vi "CheckifINorOUTIrregularForceField.vi"(0 "CenPt":dbl[](array[numeric])) -> (7 "DesiredFM_FF":dbl[](array[numeric]), 8 "Current_point":dbl[](array[numeric]), 10 "in":bool)   [LabVIEW 2017]
uses:
  <vilib>/imath/engines/lvmath2/RunTimeEngine/IndexRead/NIMS V(S).vi
  <instcachedir>/0/NIMS V(S)_0488751826AF41519A22953C041130DC.lvgen/NIMS V(S)_0488751826AF41519A22953C041130DC_000.vi
  <vilib>/imathl/engines/lvmath/Functions/Error Handling/Create Error.vi
  <vilib>/imath/engines/lvmath2/RunTimeEngine/VariableToken/NIMS_VariableToken_CondDefined.vi
  <instcachedir>/0/NIMS_VariableToken_CondDefined_6E7F1EE7F80E48298C84CF05BD736261.lvgen/NIMS_VariableToken_CondDefined_6E7F1EE7F80E48298C84CF05BD736261_004.vi
  <vilib>/imath/engines/lvmath/Functions/Error Handling/MergeErrorsWrapper.vi
  <vilib>/imath/engines/lvmath2/RunTimeEngine/NodeEndStatement/NIMS_NodeEndStatement_Output.vi
  <instcachedir>/0/NIMS_NodeEndStatement_Output_53EC0D466D134D7ABD903AC30B43404B.lvgen/NIMS_NodeEndStatement_Output_53EC0D466D134D7ABD903AC30B43404B_001.vi
  <instcachedir>/0/NIMS_NodeEndStatement_Output_53EC0D466D134D7ABD903AC30B43404B.lvgen/NIMS_NodeEndStatement_Output_53EC0D466D134D7ABD903AC30B43404B_005.vi
  <instcachedir>/0/NIMS_NodeEndStatement_Output_53EC0D466D134D7ABD903AC30B43404B.lvgen/NIMS_NodeEndStatement_Output_53EC0D466D134D7ABD903AC30B43404B_010.vi
  <vilib>/imath/engines/lvmath2/RunTimeEngine/ErrorHandling/NIMS_Finalize Error.vi
panel:
  out "z":dbl
  out "y":dbl
  out "x":dbl
  out "c":dbl
  out "b":dbl
  out "a":dbl
  out "value":dbl
  out "FX FY FZ 0 0 0":dbl[](array[numeric])
  out "Fx, Fy, Fz":dbl[](array[numeric])
  out "subarray 2":dbl[](array[numeric])
  out "Desired FM_FF":dbl[](array[numeric])
  # "Inputs"
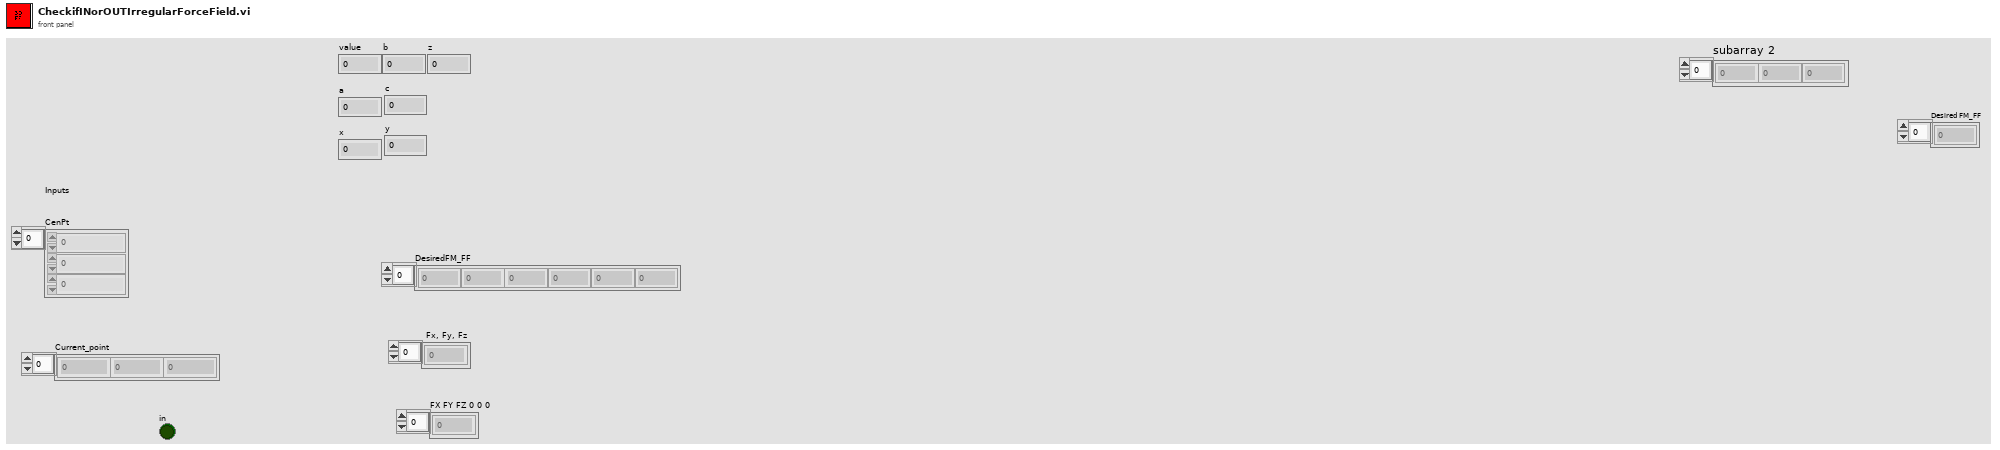
[diagram p1: front panel]
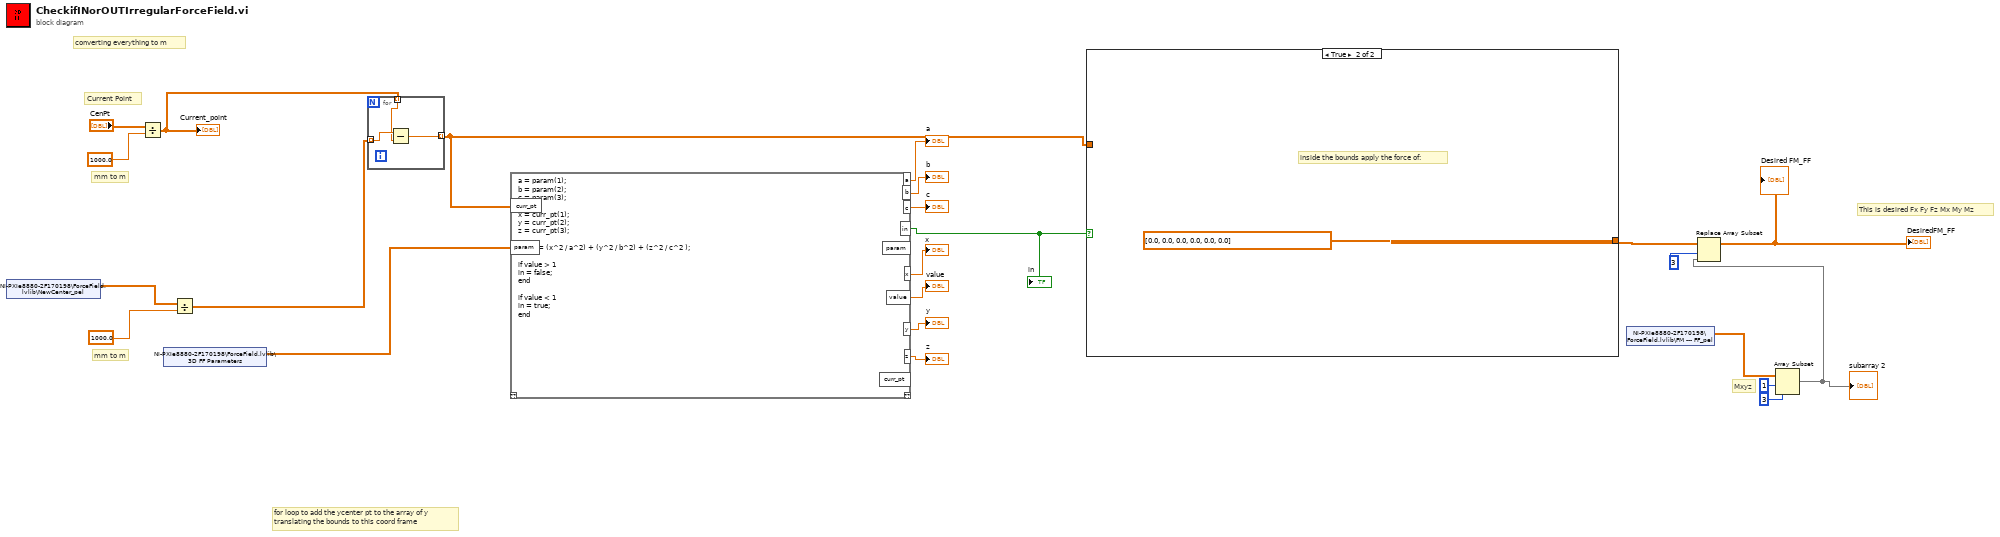
[diagram p0: block diagram]
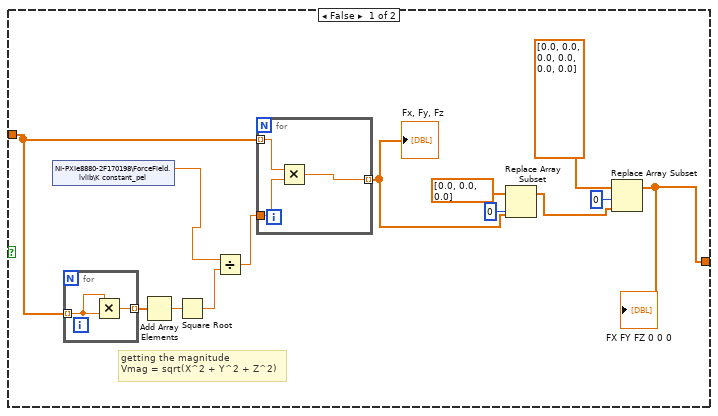
[diagram p2: hidden frame]
diagram:
  # "for loop to add the ycenter pt to the array of y\ntranslating the bounds to this coord frame"
  # "This is desired Fx Fy Fz Mx My Mz"
  # "converting everything to m"
  # "Mxyz"
  # "mm to m"
  # "Current Point"
  # "mm to m"
  n1 = shared-variable "NI-PXIe8880-2F170198\\ForceField.lvlib\\NewCenter_pel"() -> (w9:dbl[])  [unwired: 1 in, 1 out]
  n2 = Divide(x="CenPt", y=1000.0) -> (x/y=w13:dbl[])
  "Current_point" <- w13
  n3 = shared-variable "NI-PXIe8880-2F170198\\ForceField.lvlib\\3D FF Parameters"() -> (w12:dbl[])  [unwired: 1 in, 1 out]
  n4 = Divide(x=w9, y=1000.0) -> (x/y=w14:dbl[])
  n5 = for {
    tunnel: w14 -> [w25] mode=indexing
    tunnel: w13 -> [w24] mode=indexing
    tunnel: [w26] -> w11 mode=indexing
    n6 = Subtract(x=w25, y=w24) -> (x-y=w26:dbl)
  }
  n7 = mathscript code="a = param(1);\nb = param(2);\nc = param(3);\n\nx = curr_pt(1);\ny = curr_pt(2);\nz = curr_pt(3);\n\nvalue = (x^2 / a^2) + (y^2 / b^2) + (z^2 / c^2 );\n\nif value > 1\nin = false;\nend\n\nif value < 1\nin = true;\nend"("curr_pt"=w11, "param"=w12) -> ("in"=w10:bool, "value"=→"value":dbl, "a"=→"a":dbl, "b"=→"b":dbl, "c"=→"c":dbl, "x"=→"x":dbl, "y"=→"y":dbl, "z"=→"z":dbl)  [unwired: 1 in, 3 out]
  "in" <- w10
  n8 = case shown="True" w10 {
    tunnel: [w28 dbl[] [0.0, 0.0, 0.0, 0.0, 0.0, 0.0]] -> w8
    tunnel: w11 -> [w36 _]
    frame False {
      # "getting the magnitude\nVmag = sqrt(X^2 + Y^2 + Z^2)"
      n9 = shared-variable "NI-PXIe8880-2F170198\\ForceField.lvlib\\K constant_pel"() -> (w27:dbl)  [unwired: 1 in, 1 out]
      n10 = for {
        tunnel: w36 -> [w44] mode=indexing
        tunnel: [w43] -> w38 mode=indexing
        n11 = Multiply(x=w44, y=w44) -> (x*y=w43:dbl)
      }
      n12 = Add Array Elements(numeric array=w38) -> (sum=w39:dbl)
      n13 = Square Root(x=w39) -> (sqrt(x)=w37:dbl)
      n14 = Divide(x=w27, y=w37) -> (x/y=w35:dbl)
      n15 = for {
        tunnel: w36 -> [w42] mode=indexing
        tunnel: w35 -> [w41]
        tunnel: [w40] -> w32 mode=indexing
        n16 = Multiply(x=w42, y=w41) -> (x*y=w40:dbl)
      }
      "Fx, Fy, Fz" <- w32
      n17 = Replace Array Subset(array=dbl[] [0.0, 0.0, 0.0], new element=w32, index=0) -> (w29:dbl[])
      n18 = Replace Array Subset(array=dbl[] [0.0, 0.0, 0.0, 0.0, 0.0, 0.0] ("element"), new element=w29, index=0) -> (w28:dbl[])
      "FX FY FZ 0 0 0" <- w28
    }
    frame True {
      # "inside the bounds apply the force of:"
    }
  }
  n19 = shared-variable "NI-PXIe8880-2F170198\\ForceField.lvlib\\FM --- FF_pel"() -> (w18:dbl[])  [unwired: 1 in, 1 out]
  n20 = Array Subset(array=w18, index=1, length=3) -> (w15:dbl[])
  "subarray 2" <- w15
  n21 = Replace Array Subset(array=w8, new element=w15, index=3) -> (→"DesiredFM_FF" →"Desired FM_FF":dbl[])
